vi "Read Refs.vi"(11 "Base Attributes in":refnum<class "Base Attributes.lvclass">) -> (2 "Refs":refnum<class "Refs.lvclass">)   [LabVIEW 2025, in "jettl.lvlib" / "Attributes.lvlib" / "Base Attributes.lvclass"]
uses:
  Base Attributes.lvclass
  Base Attributes.lvclass/Base Attributes.ctl
  Refs/Refs.lvclass
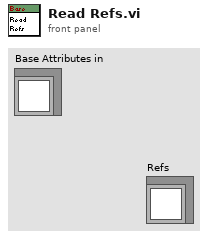
[diagram p1: front panel]
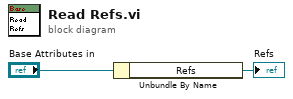
[diagram p0: block diagram]
diagram:
  n1 = Unbundle By Name("Base Attributes in") -> ("Refs"=→"Refs":refnum<class "Refs.lvclass">)
